vi "总磷总氮版本号读取.vi"(8 "Error in":errorcluster caption="Error in (no error)") -> (0 "error out":errorcluster, 3 "固件版本号":string)   [LabVIEW 2016, in "斯坦道总磷.lvlib"]
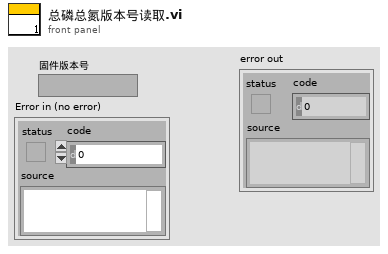
[diagram p1: front panel]
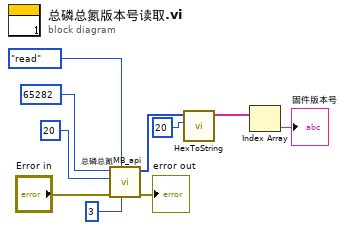
[diagram p0: block diagram]
diagram:
  n1 = call "总磷总氮MB_api.vi"("Slave ID"=u8 3, "STEP"=enum16{"open", "read", "write", "close"}."read", "Error in"="Error in", "quantity"=u16 20, "starting address"=u16 65282) -> ("error out"=→"error out":errorcluster, "Registers"=w4:u16[])  [unwired: 4 in, 1 out]
  n2 = call "HexToString.vi"("字符个数"=20, "数组"=w4) -> ("STRING"=w2:string[])  [unwired: 9 in]
  n3 = Index Array(array=w2) -> (element=→"固件版本号":string)  [unwired: 1 in]
